vi "main.vi"() -> ()   [LabVIEW 2023]
panel:
  out "Przebieg temperatur":dynamicdata(graph)
  in  "Wybor":enum32{"Symulacja", "Pomiar", "S&P"}(radio)=enum."S&P"
  in  "Dane Pomiarowe":path=path "D:/__studia/Semestr_6/SUS/_Projekt/HeatExchangerSimulation/Data/Pomiary.txt"
  in  "Zapis do pliku":bool
  in  "Ścieżka do pliku":path=path "D:/__studia/Semestr_6/SUS/_Projekt/HeatExchangerSimulation/Data/ZapisaneDane.txt"
  in  "ThStart [°C]":dbl
  in  "Spowolnienie Symulacji":dbl(slide) scale=0.5..6.0
  in  "Stop":bool
  in  "Ciecz":T1={"Thin [°C]"=20.0, "V [m3]"=0.0025, "cw [J/(kg*K)]"=4200.0, "ro [kg/m3]"=997.0, "F1 [m2/min]"=2.0, "Ph [W]"=11400.0, "Pnom [%]"=20.0, "h"=1.0}
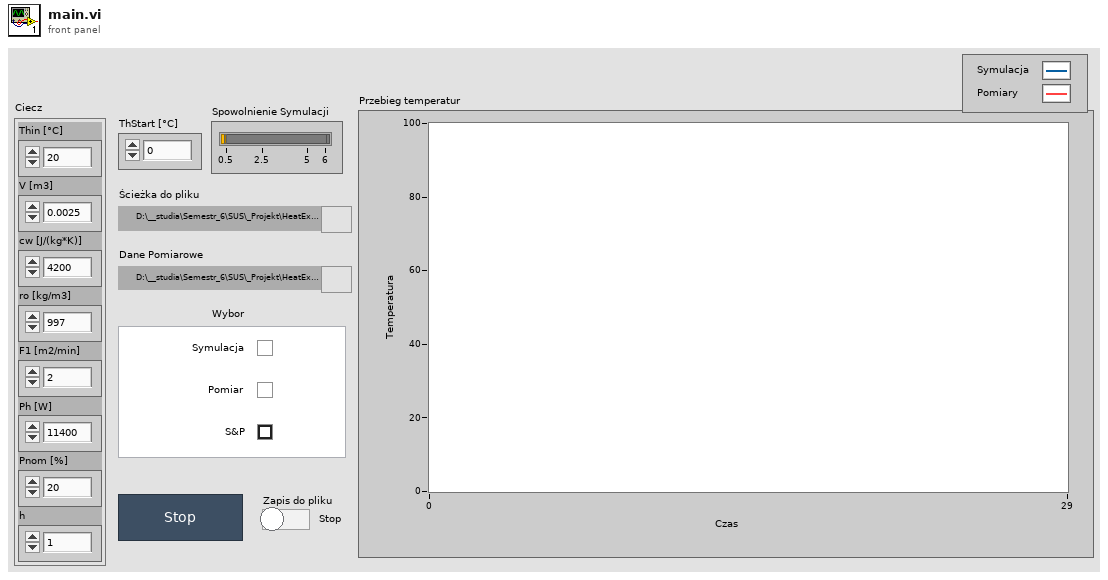
[diagram p1: front panel]
types:
  T1 = cluster{"Thin [°C]":dbl, "V [m3]":dbl, "cw [J/(kg*K)]":dbl, "ro [kg/m3]":dbl, "F1 [m2/min]":dbl, "Ph [W]":dbl, "Pnom [%]":dbl, "h":dbl}
  T2 = enum16{"open", "replace", "create", "open or create", "replace or create", "replace or create with confirmation"}
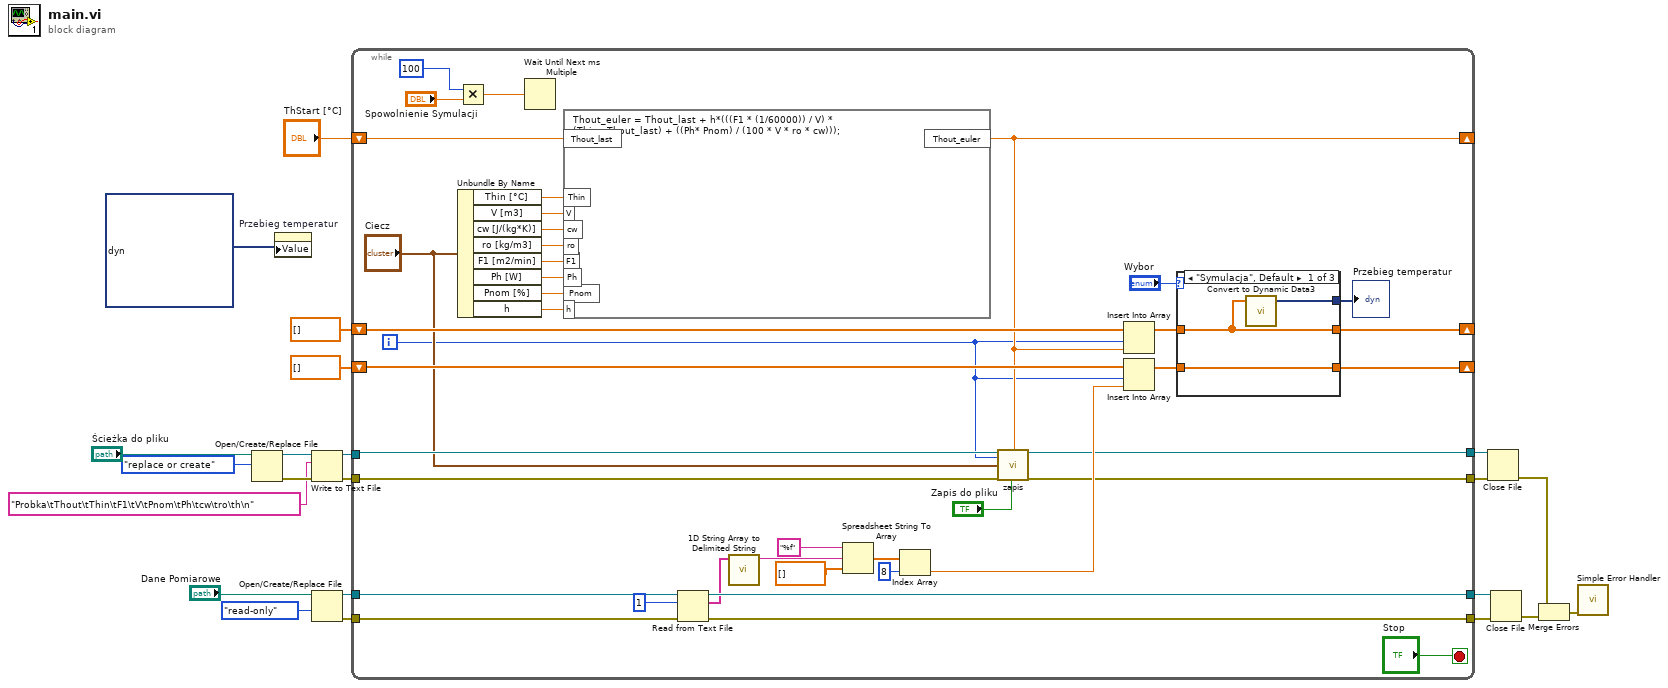
[diagram p0: block diagram]
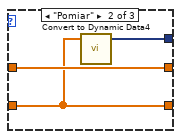
[diagram p2: hidden frame]
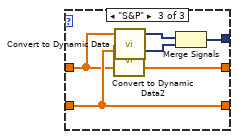
[diagram p3: hidden frame]
diagram:
  n1 = Open/Create/Replace File(file path (use dialog)="Ścieżka do pliku", operation (0:open)=T2."replace or create") -> (refnum out=w15:refnum<file>, error out=w14:errorcluster)  [unwired: 4 in, 1 out]
  n2 = property on="Przebieg temperatur" class="WFChart (strict)"("Value"=dynamicdata [{"t0"=timestamp(0 s since 1904-01-01), "dt"=1.0, "Y"=[1.3551490287444863, 2.6922294037723793, 4.011482040466567, 5.313144642004833, 6.5974517421892545, 7.86463474770455, 9.114921979812976, 10.348538715493289, 11.565707228031197, 12.7666468270686, 13.951573898118838, 15.120701941555073, 16.274241611078825, 17.412400751675595, 18.535384437064405, 19.64339500664803, 20.736632101970542, 21.815292702688755, 22.879571162064057, 23.92965924198102, 24.965746147499093, 25.98801856094359, 26.996660675542163, 27.991854228612752, 28.97377853430907, 29.942610515929434, 30.89852473779486, 31.841693436702084, 32.77228655295721, 33.6904717609956, 34.59641449959348, 35.49027800167672, 36.372223323732186, 37.24240937482691, 38.10099294524037, 38.948128734714984, 39.783969380329935, 40.60866548400335, 41.42236563962779, 42.22521645984391, 43.01736260245714, 43.7989467965022, 44.57010986795999, 45.33099076513168, 46.08172658367441, 46.82245259130324, 47.55330225216368, 48.27440725087932, 48.98589751627875, 49.687901244806184, 50.38054492361992, 51.06395335338281, 51.73824967074886, 52.40355537055002, 53.059990327687174, 53.707672818729165, 54.34671954322393, 54.97724564472543, 55.59936473154024, 56.213188897197526, 56.81882874064605, 57.41639338618192, 58.00599050311065, 58.587726325146996, 59.16170566955619, 59.72803195603993, 60.286807225370545]}, {"t0"=timestamp(0 s since 1904-01-01), "dt"=1.0, "Y"=[21.0, 21.0, 21.0, 21.0, 21.0, 21.0, 21.0, 21.0, 22.0, 22.0, 22.0, 22.0, 22.0, 22.0, 22.0, 23.0, 23.0, 23.0, 23.0, 24.0, 24.0, 24.0, 24.0, 24.0, 24.0, 25.0, 25.0, 25.0, 25.0, 25.0, 25.0, 25.0, 25.0, 25.0, 25.0, 25.0, 26.0, 26.0, 26.0, 26.0, 26.0, 26.0, 26.0, 26.0, 27.0, 27.0, 27.0, 27.0, 27.0, 27.0, 27.0, 27.0, 27.0, 27.0, 27.0, 27.0, 27.0, 27.0, 28.0, 28.0, 28.0, 28.0, 28.0, 28.0, 28.0, 28.0, 28.0]}] ("Przebieg temperatur")) -> ()  [unwired: 2 in, 2 out]
  n3 = Write to Text File(file (use dialog)=w15, text="Probka\tThout\tThin\tF1\tV\tPnom\tPh\tcw\tro\th\n", error in=w14) -> (refnum out=w12:refnum<file>, error out=w11:errorcluster)  [unwired: 1 in, 1 out]
  n4 = Open/Create/Replace File(file path (use dialog)="Dane Pomiarowe", access (0:read/write)=enum16{"read/write", "read-only", "write-only"}."read-only") -> (refnum out=w20:refnum<file>, error out=w19:errorcluster)  [unwired: 4 in, 1 out]
  n5 = while {
    shift-right: [w29] -> _
    shift-left: "ThStart [°C]" -> [w62]
    tunnel: w20 -> [w59]
    tunnel: w19 -> [w58]
    tunnel: [w51] -> w18
    tunnel: [w57] -> w17
    tunnel: w12 -> [w33]
    tunnel: w11 -> [w34]
    shift-right: [w26] -> _
    shift-left: dbl[] [] -> [w39]
    shift-right: [w25] -> _
    shift-left: dbl[] [] -> [w38]
    tunnel: [w32] -> w5
    tunnel: [w31] -> w4
    i -> [w23]
    stop <- "Stop" stop-if-true
    n6 = Multiply(x=u32 100 ("milliseconds to wait"), y="Spowolnienie Symulacji") -> (x*y=w60:dbl)
    n7 = Unbundle By Name("Ciecz") -> ("Thin [°C]"=w42:dbl, "V [m3]"=w47:dbl, "cw [J/(kg*K)]"=w43:dbl, "ro [kg/m3]"=w44:dbl, "F1 [m2/min]"=w48:dbl, "Ph [W]"=w45:dbl, "Pnom [%]"=w46:dbl, "h"=w41:dbl)
    n8 = Wait Until Next ms Multiple(millisecond multiple=w60) -> ()  [unwired: 1 out]
    n9 = formula code="Thout_euler = Thout_last + h*(((F1 * (1/60000)) / V) * \n(Thin - Thout_last) + ((Ph* Pnom) / (100 * V * ro * cw)));"("F1"=w48, "V"=w47, "Pnom"=w46, "Ph"=w45, "ro"=w44, "cw"=w43, "Thout_last"=w62, "Thin"=w42, "h"=w41) -> ("Thout_euler"=w29:dbl)
    n10 = Read from Text File(file (use dialog)=w59, count=1, error in=w58) -> (refnum out=w57:refnum<file>, text=w55:string[], error out=w51:errorcluster)  [unwired: 1 in, 1 out]
    n11 = call <vilib>:"1D String Array to Delimited String.vi"("string array"=w55) -> ("delimited string"=w54:string)  [unwired: 10 in]
    n12 = Spreadsheet String To Array(format string="%f", spreadsheet string=w54, array type (2D Dbl)=dbl[] [] ("array type (1D Dbl)")) -> (array=w49:dbl[])  [unwired: 1 in]
    n13 = Index Array(array=w49, index=8) -> (element=w37:dbl)
    n14 = call "zapis.vi"("Byte Stream File Refnum"=w33, "error in (no error)"=w34, "Ciecz in"="Ciecz", "Zapis do pliku"="Zapis do pliku", "thout"=w29, "probka"=w23) -> ("Byte Stream File Refnum 2"=w32:refnum<file>, "error out"=w31:errorcluster)  [unwired: 12 in]
    n15 = Insert Into Array(array=w39, index=w23, new element=w29) -> (w27:dbl[])
    n16 = Insert Into Array(array=w38, index=w23, new element=w37) -> (w36:dbl[])
    n17 = case shown="\"Symulacja\", Default" "Wybor" {
      tunnel: w27 -> [w64 w68 w71]
      tunnel: w36 -> [w65 w67 w72]
      tunnel: [w64 w68 w71] -> w26
      tunnel: [w65 w67 w72] -> w25
      tunnel: [w66 w69 w70] -> w24
      frame "Symulacja", Default {
        n18 = call "Convert to Dynamic Data3"("Array"=w64) -> ("Dynamic Data Type"=w66:dynamicdata)  [unwired: 3 in]
      }
      frame "Pomiar" {
        n19 = call "Convert to Dynamic Data4"("Array"=w67) -> ("Dynamic Data Type"=w69:dynamicdata)  [unwired: 3 in]
      }
      frame "S&P" {
        n20 = call "Convert to Dynamic Data2"("Array"=w72) -> ("Dynamic Data Type"=w74:dynamicdata)  [unwired: 3 in]
        n21 = call "Convert to Dynamic Data"("Array"=w71) -> ("Dynamic Data Type"=w73:dynamicdata)  [unwired: 3 in]
        n22 = Merge Signals(w73, w74) -> (w70:dynamicdata)
      }
    }
    "Przebieg temperatur" <- w24
  }
  n23 = Close File(refnum=w5, error in=w4) -> (error out=w3:errorcluster)  [unwired: 1 out]
  n24 = Close File(refnum=w17, error in=w18) -> (error out=w2:errorcluster)  [unwired: 1 out]
  n25 = Merge Errors(w3, w2) -> (w13:errorcluster)
  n26 = call <vilib>:"Simple Error Handler.vi"("error in (no error)"=w13) -> ()  [unwired: 4 in, 5 out]
